vi "InstrClose.vi"(8 "error in (no error)":errorcluster, 11 "Instruments in":refnum<class "Instruments.lvclass">) -> (0 "error out":errorcluster, 3 "Instruments out":refnum<class "Instruments.lvclass">)   [LabVIEW 2012, in "Instruments.lvclass"]
uses:
  Instruments.lvclass
  Instruments.lvclass/Instruments.ctl
  <instrlib>/Keithley 24XX/Keithley 24XX.lvlib
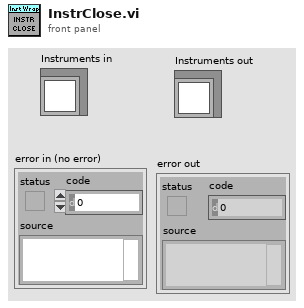
[diagram p1: front panel]
types:
  T1 = typedef "OphirRef.ctl" = cluster{"OphirComRef":refnum<k7>, "deviceHandle":i32, "Channel":i32, "SerialNumber":string, "Background Wl":dbl, "Background":dbl, "CalWl":dbl}
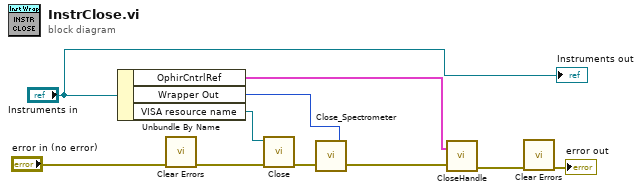
[diagram p0: block diagram]
diagram:
  n1 = Unbundle By Name("Instruments in") -> ("OphirCntrlRef"=w3:T1, "Wrapper Out"=w9:u32, "VISA resource name"=w8:refnum<visa-resource-name>)
  n2 = call <vilib>:"Clear Errors.vi"("error in (no error)"="error in (no error)") -> ("error out"=w4:errorcluster)  [unwired: 6 in]
  n3 = call <instrlib>:"Close.vi"("error in (no error)"=w4, "VISA resource name"=w8) -> ("error out"=w7:errorcluster)  [unwired: 9 in]
  n4 = call "Close_Spectrometer.vi"("Spectr* In"=w9, "error in (no error)"=w7) -> ("error out"=w2:errorcluster)  [unwired: 1 in]
  n5 = call "CloseHandle.vi"("error in (no error)"=w2, "OphirRef In"=w3) -> ("error out"=w1:errorcluster)  [unwired: 1 out]
  n6 = call <vilib>:"Clear Errors.vi"("error in (no error)"=w1) -> ("error out"=→"error out":errorcluster)  [unwired: 6 in]
  "Instruments out" <- "Instruments in"
